vi "AcquireCameraImages.vi"() -> ()   [LabVIEW 2019]
doc: "The Acquire Every Image example shows the basics of using a grab acquisition to acquire every image. A grab copies image data from driver-allocated buffers to user-allocated buffers for further processing. For performance-critical applications, it is recommended to use the Acquire Every Image (Optimized Performance) example if possible to avoid the additional overhead of an image copy. The optimized example does have some restrictions that are described in that VI. If the requirements of the optimized example are too restrictive, this one should be used instead."
uses:
  <vilib>/vision/driver/IMAQdx.llb/IMAQdx Buffer Number Mode.ctl
  <vilib>/vision/driver/NI_Vision_Acquisition_Software.lvlib
  <resource>/objmgr/imaqdx.rc
panel:
  in  "Percent of Images Reserved by Driver":dbl=50.0
  in  "Overwrite Mode":u16(ring) items=["Get Oldest"=0, "Fail"=2, "Get Newest"=3]
  in  "Simulated Processing Delay (ms)":i32
  out "Images Missed":u32
  out "Images Behind":i32
  out "Processing Frame Rate":dbl
  in  "Number of Images":u32=10
  in  "Camera Name":refnum<k21> caption="IMAQdx Session"
  out "Buffer Number":u32
  out "Image":T1(plugin-control)
  out "Acquired Frame Rate":dbl
  in  "Stop":bool
  # "Overview: Demonstrates how to acquire every image continuously using a grab acquisition.\nRequirements: Vision Acquisition Software\nInstructions:\n1. Select the Camera Name\n2. Run the VI\n3. Increase the Simulated Processing Delay to see the effect on Images Behind and Images Missed when the acquisition loop isn't executed as quickly as the camera acquires images."
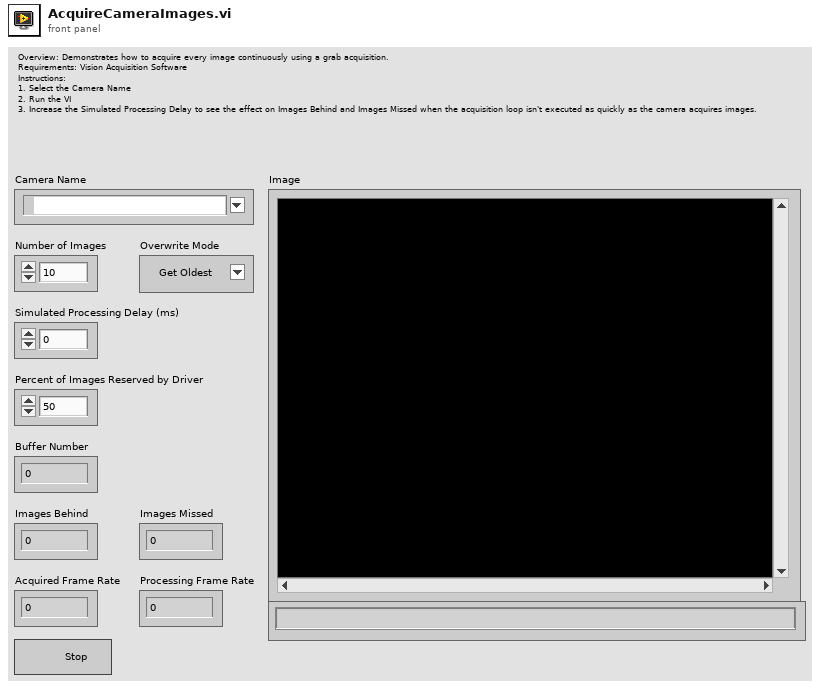
[diagram p1: front panel]
types:
  T1 = typedef "IMAQ Image.ctl" = refnum<image>
  T2 = typedef "Image Type" = u32
  T3 = typedef "IMAQdx.ctl" = refnum<k21>
  T4 = typedef "NI_Vision_Acquisition_Software.lvlib/IMAQdx Buffer Number Mode.ctl" = enum32{"Next", "Last", "Buffer Number", "Every", "Last New"}
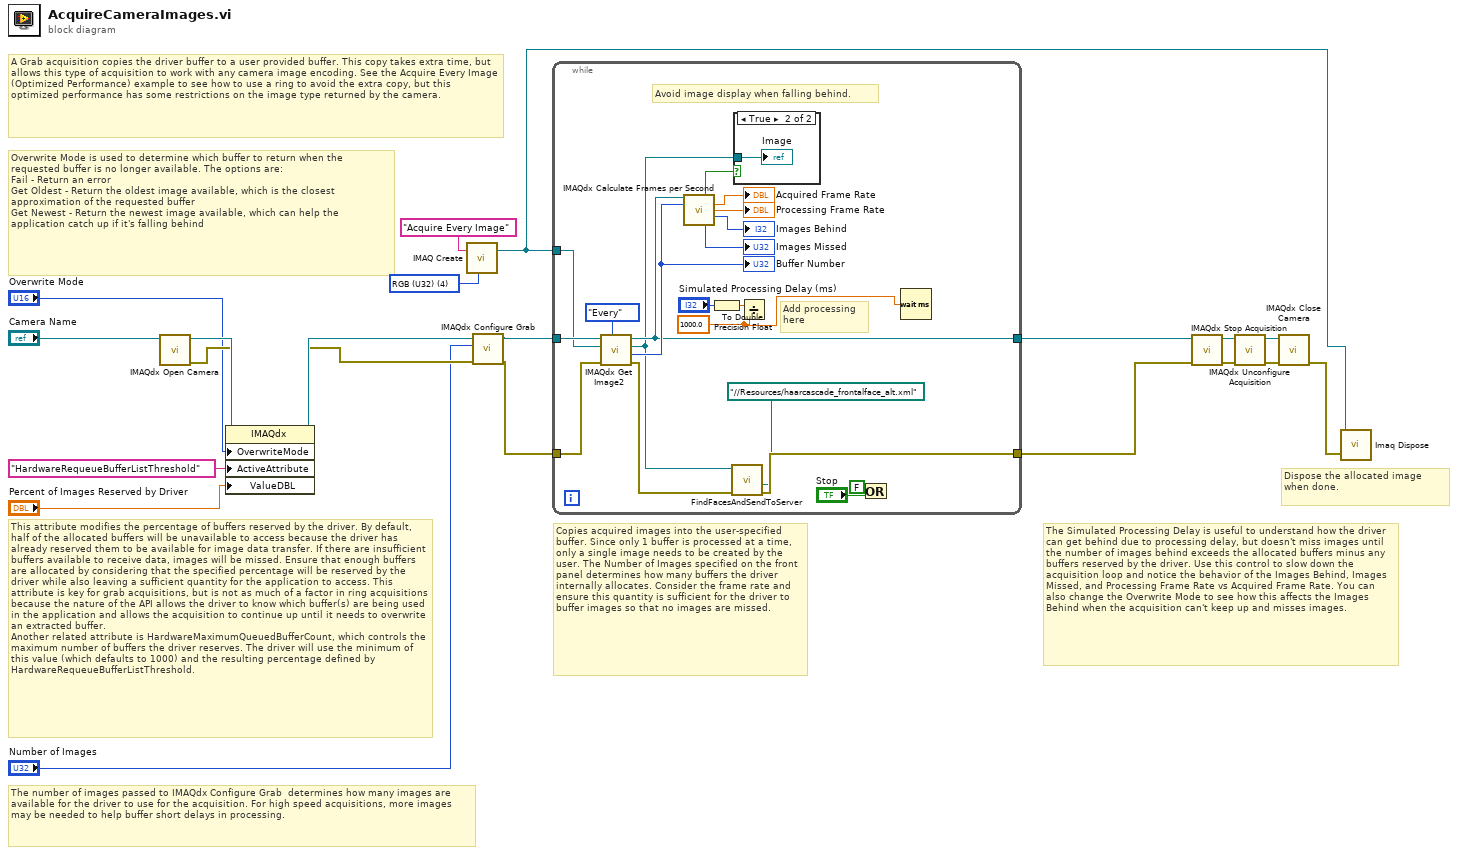
[diagram p0: block diagram]
diagram:
  w1 = T2 4 items=["Grayscale (U8)", "Grayscale (I16)", "Grayscale (SGL)", "Complex (CSG)", "RGB (U32)", "HSL (U32)", "RGB (U64)", "Grayscale (U16)"] ("Image Type")
  # "The Simulated Processing Delay is useful to understand how the driver can get behind due to processing delay, but doesn't miss images until the number of images behind exceeds the allocated buffers minus any buffers reserved by the driver. Use this control to slow down the acquisition loop and notice the behavior of the Images Behind, Images Missed, and Processing Frame Rate vs Acquired Frame Rate. You can also change the Overwrite Mode to see how this affects the Images Behind when the acquisition can't keep up and misses images."
  # "Overwrite Mode is used to determine which buffer to return when the requested buffer is no longer available. The options are:\nFail - Return an error\nGet Oldest - Return the oldest image available, which is the closest approximation of the requested buffer\nGet Newest - Return the newest image available, which can help the application catch up if it's falling behind"
  # "This attribute modifies the percentage of buffers reserved by the driver. By default, half of the allocated buffers will be unavailable to access because the driver has already reserved them to be available for image data transfer. If there are insufficient buffers available to receive data, images will be missed. Ensure that enough buffers are allocated by considering that the specified percentage will be reserved by the driver while also leaving a sufficient quantity for the application to access. This attribute is key for grab acquisitions, but is not as much of a factor in ring acquisitions because the nature of the API allows the driver to know which buffer(s) are being used in the application and allows the acquisition to continue up until it needs to overwrite an extracted buffer.\nAnother related attribute is HardwareMaximumQueuedBufferCount, which controls the maximum number of buffers the driver reserves. The driver will use the minimum of this value (which defaults to 1000) and the resulting percentage defined by HardwareRequeueBufferListThreshold."
  # "The number of images passed to IMAQdx Configure Grab  determines how many images are available for the driver to use for the acquisition. For high speed acquisitions, more images may be needed to help buffer short delays in processing."
  # "Dispose the allocated image when done."
  # "A Grab acquisition copies the driver buffer to a user provided buffer. This copy takes extra time, but allows this type of acquisition to work with any camera image encoding. See the Acquire Every Image (Optimized Performance) example to see how to use a ring to avoid the extra copy, but this optimized performance has some restrictions on the image type returned by the camera."
  # "Copies acquired images into the user-specified buffer. Since only 1 buffer is processed at a time, only a single image needs to be created by the user. The Number of Images specified on the front panel determines how many buffers the driver internally allocates. Consider the frame rate and ensure this quantity is sufficient for the driver to buffer images so that no images are missed."
  n1 = call <vilib>:"IMAQdx Open Camera.vi"("Session In"="Camera Name") -> ("error out"=w14:errorcluster, "Session Out"=w15:T3)  [unwired: 2 in, 7 out]
  n2 = property class="IMAQdx"(reference=w15, error in=w14, "OverwriteMode"="Overwrite Mode", "ActiveAttribute"="HardwareRequeueBufferListThreshold", "ValueDBL"="Percent of Images Reserved by Driver") -> (reference out=w4:T3, error out=w3:errorcluster)
  n3 = call "IMAQ Create"("Image Name"="Acquire Every Image", "Image Type"=w1) -> ("New Image"=w9:T1)  [unwired: 2 in, 2 out]
  n4 = call <vilib>:"IMAQdx Configure Grab.vi"("error in"=w3, "Number of Buffers"="Number of Images", "Session In"=w4) -> ("error out"=w5:errorcluster, "Session Out"=w6:T3)  [unwired: 7 in]
  n5 = while {
    tunnel: [w31] -> w11
    tunnel: w5 -> [w36]
    tunnel: w6 -> [w35]
    tunnel: [w26] -> w10
    tunnel: w9 -> [w33]
    stop <- w42 stop-if-true
    w23 = 1000.0 ("y")
    # "Avoid image display when falling behind."
    # "Add processing here"
    n6 = call <vilib>:"IMAQdx Get Image2.vi"("Buffer Number Mode (Next)"=IMAQdx_Buffer_Number_Mode."Every" ("Buffer Number Mode"), "error in"=w36, "Image In"=w33, "Session In"=w35) -> ("error out"=w27:errorcluster, "Buffer Number Out"=w32:u32, "Image Out"=w22:T1, "Session Out"=w31:T3)  [unwired: 4 in]
    "Buffer Number" <- w32
    n7 = call <vilib>:"IMAQdx Calculate Frames per Second.vi"("Session In"=w31, "Buffer Number"=w32) -> ("Update Display"=w38:bool, "Acquired Frames per Second"=→"Acquired Frame Rate":dbl, "Processed Frames per Second"=→"Processing Frame Rate":dbl, "Images Behind"=→"Images Behind":i32, "Images Missed"=→"Images Missed":u32)  [unwired: 7 in, 2 out]
    n8 = To Double Precision Float(number="Simulated Processing Delay (ms)") -> (double precision float=w28:dbl)
    n9 = call "FindFacesAndSendToServer.vi"("error in"=w27, "Face Cascade Path"=path "../../Resources/haarcascade_frontalface_alt.xml", "Image In"=w22) -> ("error out"=w26:errorcluster)  [unwired: 8 in]
    n10 = case shown="True" w38 {
      tunnel: w22 -> [_ w43]
      frame False {
      }
      frame True {
        "Image" <- w43
      }
    }
    n11 = Divide(x=w28, y=w23) -> ()  [unwired: 1 out]
    n12 = Or(x=FALSE, y="Stop") -> (x .or. y?=w42:bool)
    n13 = Wait (ms)(milliseconds to wait=w23) -> ()  [unwired: 1 out]
  }
  n14 = call <vilib>:"IMAQdx Stop Acquisition.vi"("error in"=w10, "Session In"=w11) -> ("error out"=w17:errorcluster, "Session Out"=w18:T3)  [unwired: 8 out]
  n15 = call <vilib>:"IMAQdx Unconfigure Acquisition.vi"("error in"=w17, "Session In"=w18) -> ("error out"=w20:errorcluster, "Session Out"=w19:T3)  [unwired: 8 out]
  n16 = call <vilib>:"IMAQdx Close Camera.vi"("error in"=w20, "Session In"=w19) -> ("error out"=w16:errorcluster)  [unwired: 9 out]
  n17 = call "Imaq Dispose"("Image"=w9, "error in (no error)"=w16) -> ()  [unwired: 4 in, 1 out]
